vi "解析坐标.vi"(8 "线号":string, 10 "匹配字符":string="J", 11 "解析数组":string[](array[string])) -> (1 "编码数值":i32, 2 "进出线选项":T1, 3 "坐标xy顺序":string[](array[string]))   [LabVIEW 2014]
uses:
  Global.vi
  <vilib>/vision/NI_Vision_Development_Module.lvlib
panel:
  out "数组":string[](array[string])
  out "数组输出 2":string[](array[string])
  out "数组输出":string[](array[string])
  out "x >= 0?":bool
  # "第二象限顺/逆"
  # "第一象限顺/逆"
  # "第三象限顺/逆"
  # "第四象限顺/逆"
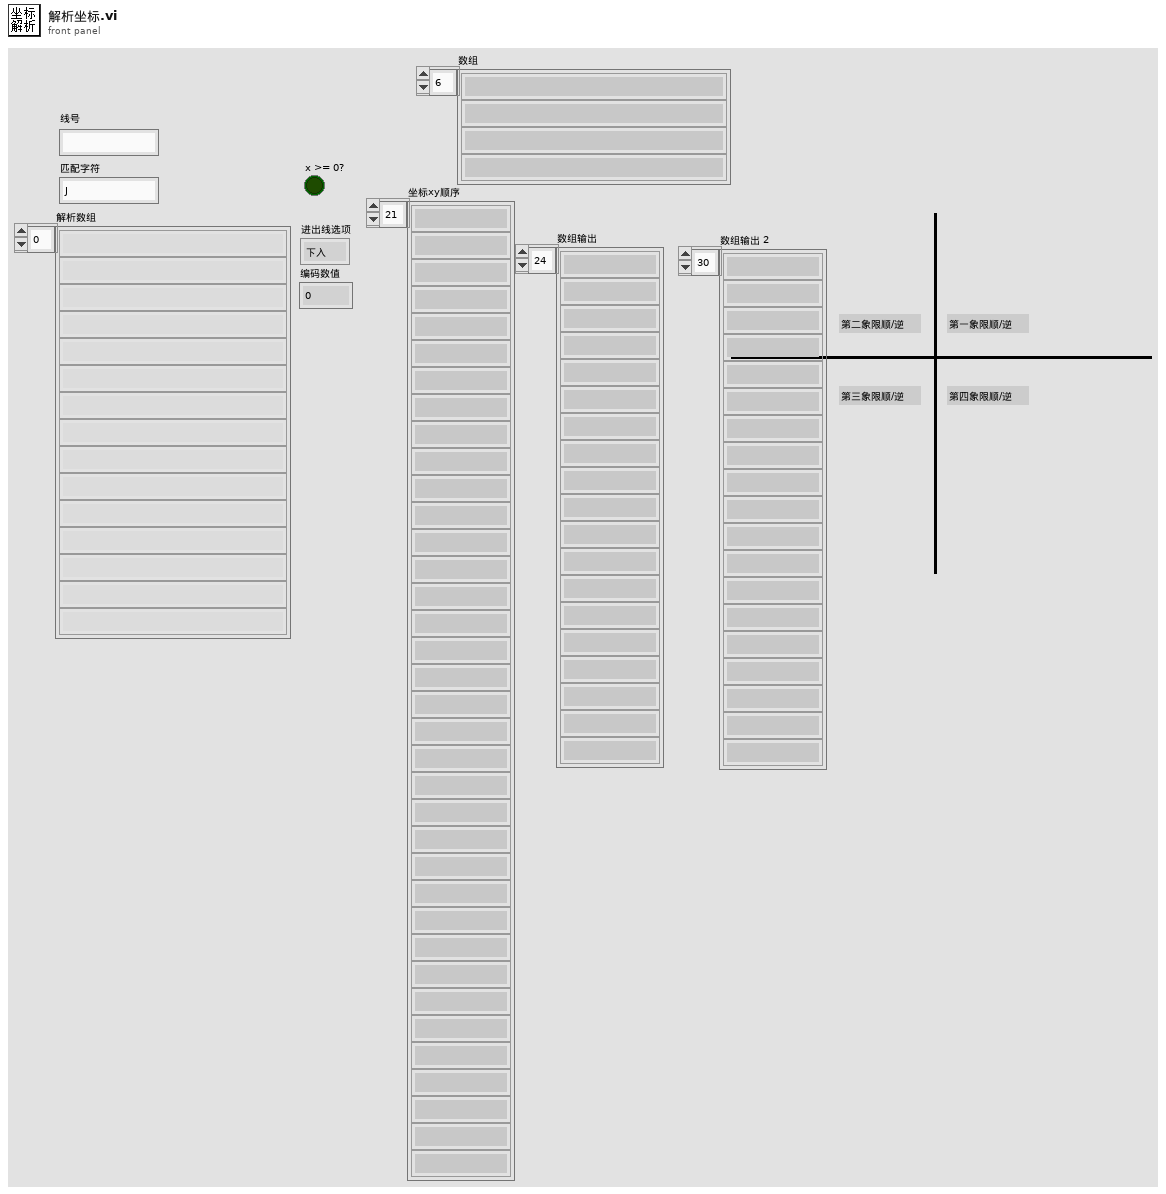
[diagram p1: front panel]
types:
  T1 = typedef "进出线选项.ctl" = enum16{"下入", "上入", "下出", "上出"}
  T2 = cluster{"Center":cluster{"X":sgl, "Y":sgl}, "Radius":dbl}
  T3 = typedef "XYPos.ctl" = cluster{"X":dbl, "Y":dbl}
  T4 = typedef "mark规格.ctl" = cluster{"X下限":dbl, "X上限":dbl, "Y下限":dbl, "Y 上限":dbl, "angle下限":dbl, "angle上限":dbl}
  T5 = cluster{"甩线补偿值":cluster{"下边":dbl, "距离上边":dbl, "左边":dbl, "右边":dbl}, "补偿甩线坐标偏移":T3, "mark点模组补偿":T3, "出线补偿值":dbl, "mark规格":T4}
  T6 = cluster{"下边":dbl, "距离上边":dbl, "左边":dbl, "右边":dbl}
  T7 = cluster{"result string":dbl, "result string":dbl}
  T8 = cluster{"result string":dbl, "result string":dbl}[]
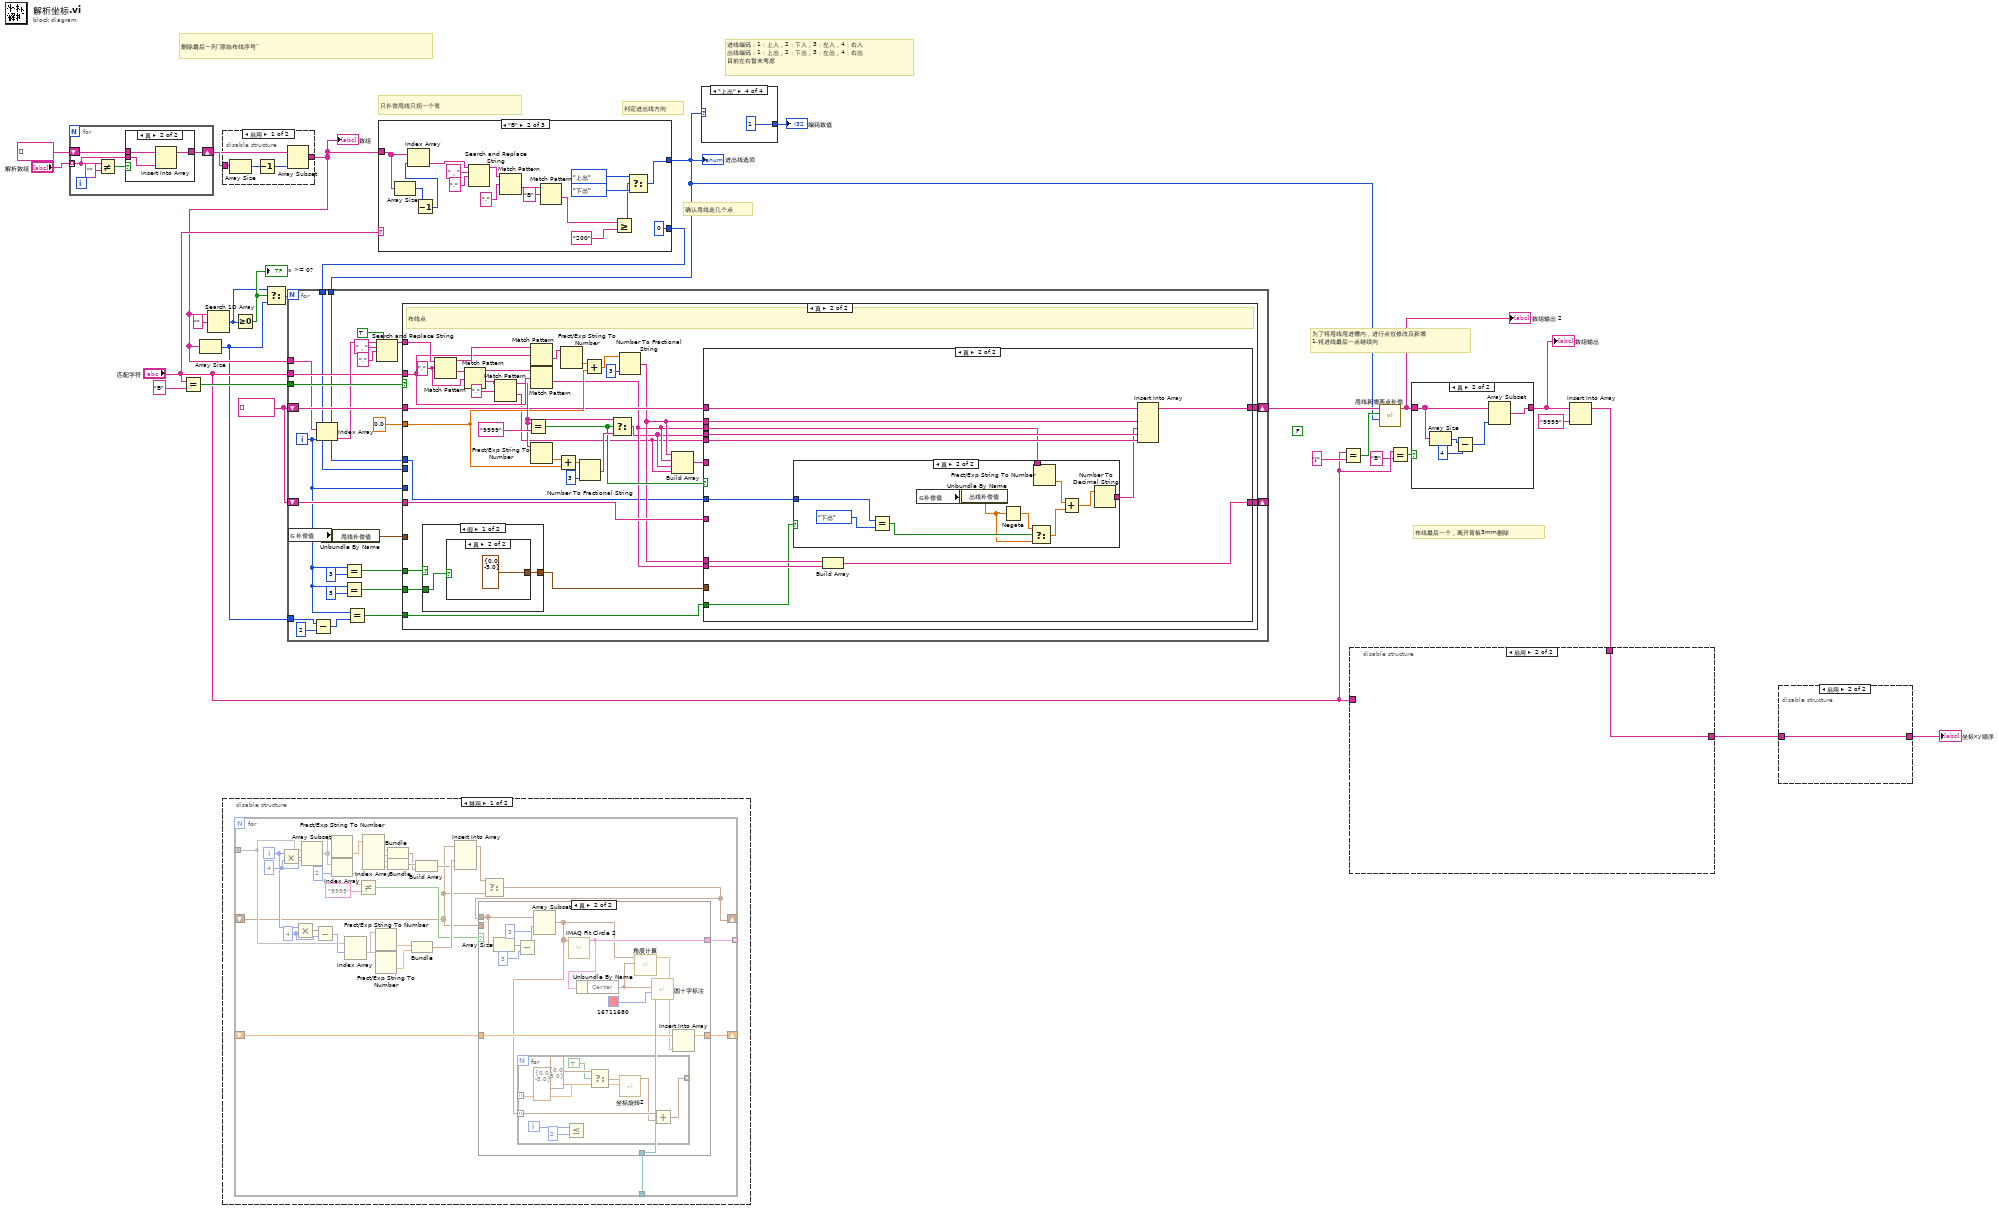
[diagram p0: block diagram]
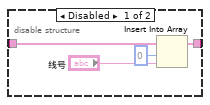
[diagram p3: hidden frame]
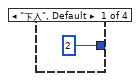
[diagram p5: hidden frame]
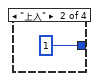
[diagram p6: hidden frame]
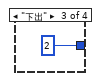
[diagram p7: hidden frame]
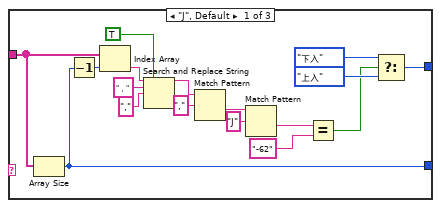
[diagram p8: hidden frame]
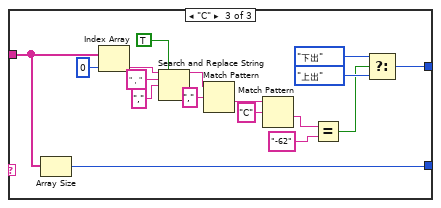
[diagram p9: hidden frame]
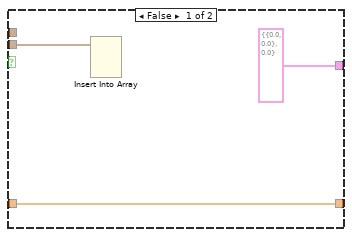
[diagram p11: hidden frame]
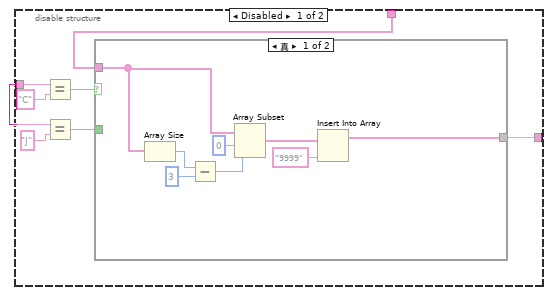
[diagram p13: hidden frame]
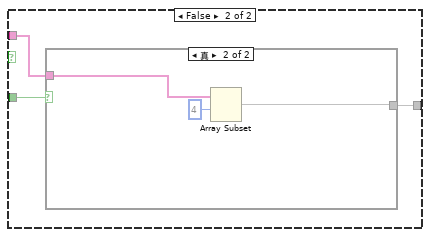
[diagram p14: hidden frame]
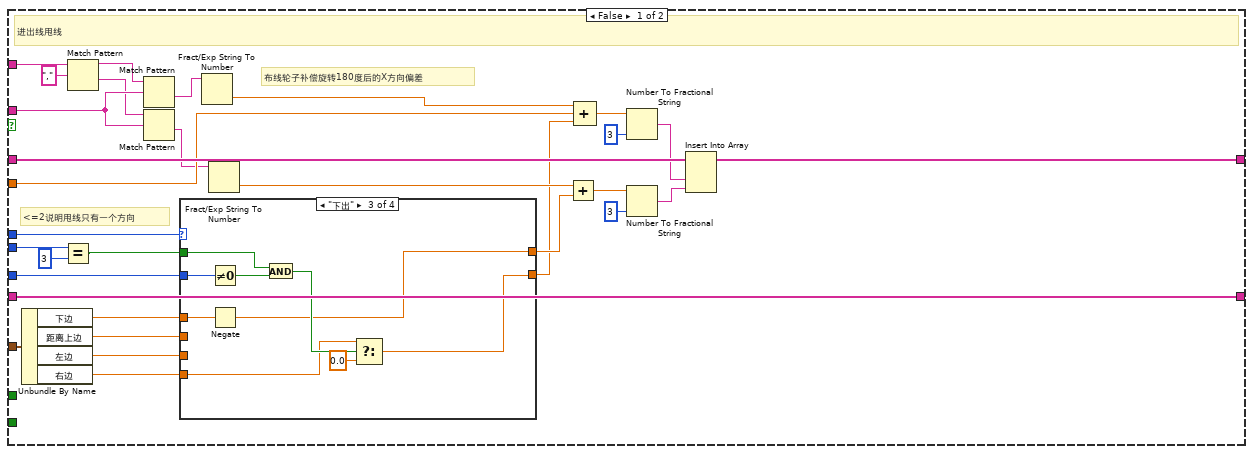
[diagram p16: hidden frame]
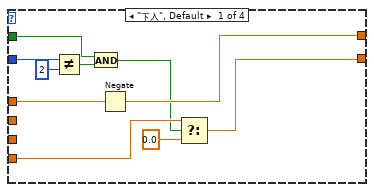
[diagram p17: hidden frame]
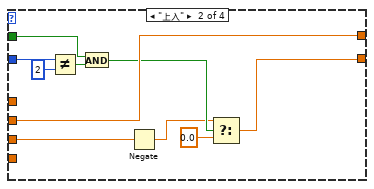
[diagram p18: hidden frame]
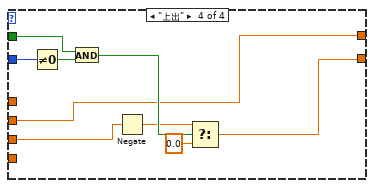
[diagram p19: hidden frame]
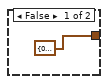
[diagram p20: hidden frame]
diagram:
  (unwired) FALSE
  w19 = string[] []
  # "删除最后一列“原始布线序号”"
  # "布线最后一个，离开背板3mm删除"
  # "为了将甩线甩进槽内，进行点位修改及新增\n1.将进线最后一点继续向"
  # "进线编码：1：上入，2：下入，3：左入，4：右入\n出线编码：1：上出，2：下出，3：左出，4：右出\n目前左右暂未考虑"
  # "确认甩线走几个点"
  # "判定进出线方向"
  # "只补偿甩线只拐一个弯"
  n1 = for {
    tunnel: "解析数组" -> [w28] mode=indexing
    shift-right: [w31] -> w5
    shift-left: string[] [] -> [w32]
    n2 = Not Equal?(x=w28, y="") -> (x != y?=w29:bool)
    n3 = case shown="真" w29 {
      tunnel: w32 -> [w33 w36]
      tunnel: [w33 w35] -> w31
      tunnel: w28 -> [_ w34]
      frame False {
      }
      frame True {
        n4 = Insert Into Array(array=w36, new element=w34) -> (w35:string[])  [unwired: 1 in]
      }
    }
  }
  n5 = Equal?(x="匹配字符", y="B") -> (x = y?=w26:bool)
  n6 = disable-structure shown="启用" {
    disable-tunnel: w5 -> [w40 w41]
    disable-tunnel: [w39 w41] -> w4
    frame Enabled {
      n7 = Array Size(array=w40) -> (size(s)=w38:i32)
      n8 = Decrement(x=w38) -> (x-1=w37:i32)
      n9 = Array Subset(array=w40, length=w37) -> (w39:string[])  [unwired: 1 in]
    }
    frame Disabled {
    }
  }
  "数组" <- w4
  n10 = Array Size(array=w4) -> (size(s)=w1:i32)
  n11 = Search 1D Array(1D array=w4, element="" ("元素")) -> (index of element=w23:i32)  [unwired: 1 in]
  n12 = disable-structure shown="禁用" {
    frame Disabled {
      n13 = for {
        tunnel: _ -> [w51]
        shift-right: [w46] -> _
        shift-left: _ -> [w42]
        tunnel: [w48] -> _ mode=indexing
        tunnel: _ -> [w45]
        shift-right: [w43] -> _
        shift-left: _ -> [w44]
        i -> [w52]
        w55 = 4 ("y")
        w72 = 4 ("y")
        n14 = Multiply(x=w52, y=w72) -> (x*y=w73:i32)
        n15 = Multiply(x=w52, y=w55) -> (x*y=w53:i32)
        n16 = Array Subset(array=w51, index=w73, length=w72) -> (w67:void[])
        n17 = Subtract(x=w53, y=w55) -> (x-y=w54:i32)
        n18 = Fract/Exp String To Number(string=w67) -> (number=w64:dbl[])  [unwired: 3 in, 1 out]
        n19 = Index Array(array=w67, index=2 ("索引")) -> (element=w70)
        n20 = Index Array(array=w51, index #1=w54) -> (element #1=w57, element #2=w58)  [unwired: 1 in]
        n21 = Not Equal?(x=w70, y="9999") -> (x != y?=w47:bool)
        n22 = Index Array(array=w64) -> (element #1=w66:dbl, element #2=w65:dbl, element #3=w63:dbl, element #4=w62:dbl)  [unwired: 4 in]
        n23 = Fract/Exp String To Number(string=w57) -> (number=w56:dbl)  [unwired: 3 in, 1 out]
        n24 = Fract/Exp String To Number(string=w58) -> (number=w59:dbl)  [unwired: 3 in, 1 out]
        n25 = Bundle(w66, w65) -> (w60:cluster{dbl, dbl})  [unwired: 1 in]
        n26 = Bundle(w63, w62) -> (w61:cluster{dbl, dbl})  [unwired: 1 in]
        n27 = Bundle(w56, w59) -> (w50:cluster{dbl, dbl})  [unwired: 1 in]
        n28 = Build Array(w61, w60) -> (w49:cluster{dbl, dbl}[])
        n29 = Insert Into Array(array=w42, new element #1=w50, new element #2=w49) -> (w68:cluster{dbl, dbl}[])  [unwired: 1 in]
        n30 = Select(t=w68, f=w42) -> (s? t:f=w46:cluster{dbl, dbl}[])  [unwired: 1 in]
        n31 = case shown="真" w47 {
          tunnel: [T2 {"Center"={"X"=0.0, "Y"=0.0}, "Radius"=0.0} ("Circle") w83] -> w48
          tunnel: w46 -> [_ w89]
          tunnel: w45 -> [_ w84]
          tunnel: w44 -> [w75 w80]
          tunnel: [w75 w79] -> w43
          tunnel: w42 -> [w74 _]
          frame False {
            n32 = Insert Into Array(array=w74) -> ()  [unwired: 3 in, 1 out]
          }
          frame True {
            n33 = Array Size(array=w89) -> (size(s)=w88:i32)
            n34 = Subtract(x=w88, y=3) -> (x-y=w86:i32)
            n35 = Array Subset(array=w89, index=w86, length=3 ("长度")) -> (w77:cluster{dbl, dbl}[])
            n36 = for {
              tunnel: w77 -> [w98] mode=indexing
              tunnel: _ -> [w99] mode=indexing
              tunnel: [w96] -> _ mode=indexing
              i -> [w95]
              n37 = Less Or Equal?(x=w95, y=2) -> ()  [unwired: 1 out]
              n38 = Select(t=cluster{"X":dbl, "Y":dbl} {"X"=0.0, "Y"=5.0} ("y"), s=TRUE, f=cluster{"X":dbl, "Y":dbl} {"X"=0.0, "Y"=-5.0} ("y")) -> (s? t:f=w92:cluster{"X":dbl, "Y":dbl})
              n39 = call "坐标旋转2.vi"("旋转角度(单位弧度)"=w99, "dtx,dty In"=w92) -> ("dtx,dty Out"=w97:cluster{"X":dbl, "Y":dbl})  [unwired: 9 in]
              n40 = Add(x=w98, y=w97) -> (x+y=w96:cluster{dbl, dbl})
            }
            n41 = call "IMAQ Fit Circle 2"("Radial Points"=w77) -> ("Circle"=w83:T2)  [unwired: 5 in, 5 out]
            n42 = Unbundle By Name(w83) -> ("Center"=w81:cluster{"X":sgl, "Y":sgl})
            n43 = call "角度计算.vi"("远心坐标"=w81, "圆弧上三个点坐标"=w77) -> ("Angle"=w78:dbl[])  [unwired: 9 in]
            n44 = call "圆十字标注.vi"("Color"=u32 16711680, "簇"=w81, "引用句柄输入"=w84) -> ()  [unwired: 8 in, 1 out]
            n45 = Insert Into Array(array=w80, new element=w78) -> (w79:dbl[])  [unwired: 1 in]
          }
        }
      }
    }
    frame Enabled {
    }
  }
  n46 = Greater Or Equal To 0?(x=w23) -> (x >= 0?=w24:bool)
  "x >= 0?" <- w24
  n47 = Select(t=w23, s=w24, f=w1) -> (s? t:f=w22:i32)
  n48 = case shown="\"B\"" "匹配字符" {
    tunnel: w4 -> [w107 w128 w150]
    tunnel: [w103 w120 w139] -> w11
    tunnel: [w100 0 w135] -> w16
    frame "J", Default {
      n49 = Array Size(array=w107) -> (size(s)=w100:i32)
      n50 = Decrement(x=w100) -> (x-1=w116:i32)
      n51 = Index Array(array=w107, index=w116) -> (element=w113:string)
      n52 = Search and Replace String(replace all?=TRUE ("替换全部？(F)"), input string=w113, search string="，" ("搜索字符串"), replace string="," ("替换字符串(\"\")")) -> (result string=w111:string)  [unwired: 4 in, 3 out]
      n53 = Match Pattern(string=w111, regular expression="," ("正则表达式")) -> (after substring=w109:string)  [unwired: 1 in, 3 out]
      n54 = Match Pattern(string=w109, regular expression="J" ("正则表达式")) -> (after substring=w101:string)  [unwired: 1 in, 3 out]
      n55 = Equal?(x=w101, y="-62") -> (x = y?=w102:bool)
      n56 = Select(t=进出线选项."下入", s=w102, f=进出线选项."上入") -> (s? t:f=w103:T1)
    }
    frame "B" {
      n57 = Array Size(array=w128) -> (size(s)=w118:i32)
      n58 = Decrement(x=w118) -> (x-1=w117:i32)
      n59 = Index Array(array=w128, index=w117) -> (element=w127:string)
      n60 = Search and Replace String(input string=w127, search string="，" ("搜索字符串"), replace string="," ("替换字符串(\"\")")) -> (result string=w125:string)  [unwired: 5 in, 3 out]
      n61 = Match Pattern(string=w125, regular expression="," ("正则表达式")) -> (after substring=w130:string)  [unwired: 1 in, 3 out]
      n62 = Match Pattern(string=w130, regular expression="B" ("正则表达式")) -> (after substring=w119:string)  [unwired: 1 in, 3 out]
      n63 = Greater Or Equal?(x=w119, y="200") -> (x >= y?=w121:bool)
      n64 = Select(t=进出线选项."上出", s=w121, f=进出线选项."下出") -> (s? t:f=w120:T1)
    }
    frame "C" {
      n65 = Array Size(array=w150) -> (size(s)=w135:i32)
      n66 = Index Array(array=w150, index=0 ("索引")) -> (element=w147:string)
      n67 = Search and Replace String(replace all?=TRUE ("替换全部？(F)"), input string=w147, search string="，" ("搜索字符串"), replace string="," ("替换字符串(\"\")")) -> (result string=w145:string)  [unwired: 4 in, 3 out]
      n68 = Match Pattern(string=w145, regular expression="," ("正则表达式")) -> (after substring=w143:string)  [unwired: 1 in, 3 out]
      n69 = Match Pattern(string=w143, regular expression="C" ("正则表达式")) -> (after substring=w137:string)  [unwired: 1 in, 3 out]
      n70 = Equal?(x=w137, y="-62") -> (x = y?=w136:bool)
      n71 = Select(t=进出线选项."下出", s=w136, f=进出线选项."上出") -> (s? t:f=w139:T1)
    }
  }
  "进出线选项" <- w11
  n72 = for {
    N: w22 -> [_]
    tunnel: w4 -> [w167]
    tunnel: "匹配字符" -> [w168]
    shift-right: [w175] -> w13
    shift-left: w19 -> [w176]
    tunnel: w26 -> [w174]
    shift-right: [w165] -> _
    shift-left: w19 -> [w166]
    tunnel: w11 -> [w160]
    tunnel: w16 -> [w159]
    tunnel: w1 -> [w155]
    i -> [w157]
    n73 = global read "Global.vi" "补偿值"() -> (w152:T5)
    n74 = Subtract(x=w155, y=2) -> (x-y=w154:i32)
    n75 = Index Array(array=w167, index=w157) -> (element=w169:string)
    n76 = Unbundle By Name(w152) -> ("甩线补偿值"=w151:T6)
    n77 = Equal?(x=w157, y=3) -> (x = y?=w163:bool)
    n78 = Equal?(x=w157, y=5) -> (x = y?=w161:bool)
    n79 = Equal?(x=w157, y=w154) -> (x = y?=w156:bool)
    n80 = Search and Replace String(replace all?=TRUE ("替换全部？(F)"), input string=w169, search string="，" ("搜索字符串"), replace string="," ("替换字符串(\"\")")) -> (result string=w171:string)  [unwired: 4 in, 3 out]
    n81 = case shown="真" w174 {
      tunnel: w168 -> [w207 w272]
      tunnel: w171 -> [w206 w279]
      tunnel: w176 -> [w202 w255]
      tunnel: [w177 w256] -> w175
      tunnel: 0.0 -> [w197 w261]
      tunnel: w166 -> [w195 w258]
      tunnel: [w195 w259] -> w165
      tunnel: w163 -> [_ w250]
      tunnel: w161 -> [_ w249]
      tunnel: w151 -> [w189 _]
      tunnel: w160 -> [w188 w247]
      tunnel: w159 -> [w180 _]
      tunnel: w157 -> [w183 _]
      tunnel: w156 -> [_ w246]
      frame False {
        # "<=2说明甩线只有一个方向"
        # "布线轮子补偿旋转180度后的X方向偏差"
        # "进出线甩线"
        n82 = Unbundle By Name(w189) -> ("下边"=w187:dbl, "距离上边"=w186:dbl, "左边"=w185:dbl, "右边"=w184:dbl)
        n83 = Equal?(x=w180, y=3) -> (x = y?=w178:bool)
        n84 = Match Pattern(string=w206, regular expression="," ("正则表达式")) -> (before substring=w204:string, after substring=w203:string)  [unwired: 1 in, 2 out]
        n85 = Match Pattern(string=w204, regular expression=w207) -> (after substring=w196:string)  [unwired: 1 in, 3 out]
        n86 = Match Pattern(string=w203, regular expression=w207) -> (after substring=w191:string)  [unwired: 1 in, 3 out]
        n87 = case shown="\"下出\"" w188 {
          tunnel: w178 -> [w210 w221 w230 w237]
          tunnel: w187 -> [w217 _ w231 _]
          tunnel: w186 -> [_ w226 _ w240]
          tunnel: w185 -> [_ w224 _ w242]
          tunnel: w184 -> [w213 _ w235 _]
          tunnel: w183 -> [w209 w219 w229 w239]
          tunnel: [w216 w226 w232 w240] -> w182
          tunnel: [w215 w227 w233 w243] -> w181
          frame "下入", Default {
            n88 = Not Equal?(x=w209, y=2 ("x")) -> (x != y?=w214:bool)
            n89 = And(x=w210, y=w214) -> (x .and. y?=w211:bool)
            n90 = Negate(x=w217) -> (-x=w216:dbl)
            n91 = Select(t=w213, s=w211, f=0.0 ("t")) -> (s? t:f=w215:dbl)
          }
          frame "上入" {
            n92 = Not Equal?(x=w219, y=2 ("x")) -> (x != y?=w218:bool)
            n93 = And(x=w221, y=w218) -> (x .and. y?=w225:bool)
            n94 = Negate(x=w224) -> (-x=w222:dbl)
            n95 = Select(t=w222, s=w225, f=0.0 ("t")) -> (s? t:f=w227:dbl)
          }
          frame "下出" {
            n96 = Not Equal To 0?(x=w229) -> (x != 0?=w228:bool)
            n97 = Negate(x=w231) -> (-x=w232:dbl)
            n98 = And(x=w230, y=w228) -> (x .and. y?=w236:bool)
            n99 = Select(t=w235, s=w236, f=0.0) -> (s? t:f=w233:dbl)
          }
          frame "上出" {
            n100 = Not Equal To 0?(x=w239) -> (x != 0?=w238:bool)
            n101 = And(x=w237, y=w238) -> (x .and. y?=w245:bool)
            n102 = Negate(x=w242) -> (-x=w241:dbl)
            n103 = Select(t=w241, s=w245, f=0.0) -> (s? t:f=w243:dbl)
          }
        }
        n104 = Fract/Exp String To Number(string=w196) -> (number=w201:dbl)  [unwired: 3 in, 1 out]
        n105 = Fract/Exp String To Number(string=w191) -> (number=w192:dbl)  [unwired: 3 in, 1 out]
        n106 = Add(x=w192, y=w182) -> (x+y=w193:dbl)
        n107 = Compound Arithmetic op=ADD(w201, w197, w181) -> (w200:dbl)
        n108 = Number To Fractional String(number=w200, precision (6)=i16 3 ("精度(6)")) -> (F-format string=w198:string)  [unwired: 2 in]
        n109 = Number To Fractional String(number=w193, precision (6)=i16 3 ("精度(6)")) -> (F-format string=w190:string)  [unwired: 2 in]
        n110 = Insert Into Array(array=w202, new element #1=w198, new element #2=w190) -> (w177:string[])  [unwired: 1 in]
      }
      frame True {
        w276 = "," ("正则表达式")
        # "布线点"
        n111 = case shown="假" w250 {
          tunnel: w249 -> [w281 _]
          tunnel: [w280 cluster{"X":dbl, "Y":dbl} {"X"=0.0, "Y"=5.0} ("y")] -> w248
          frame False {
            n112 = case shown="真" w281 {
              tunnel: [cluster{"X":dbl, "Y":dbl} {"X"=0.0, "Y"=-5.0} ("y") cluster{"X":dbl, "Y":dbl} {"X"=0.0, "Y"=-5.0} ("y")] -> w280
              frame False {
              }
              frame True {
              }
            }
          }
          frame True {
          }
        }
        n113 = Match Pattern(string=w279, regular expression=w276) -> (before substring=w274:string, after substring=w278:string)  [unwired: 1 in, 2 out]
        n114 = Match Pattern(string=w278, regular expression=w276) -> (before substring=w273:string, after substring=w277:string)  [unwired: 1 in, 2 out]
        n115 = Match Pattern(string=w277, regular expression="," ("正则表达式")) -> (before substring=w263:string, after substring=w251:string)  [unwired: 1 in, 2 out]
        n116 = Equal?(x=w263, y="9999") -> (x = y?=w260:bool)
        n117 = Match Pattern(string=w274, regular expression=w272) -> (after substring=w271:string)  [unwired: 1 in, 3 out]
        n118 = Match Pattern(string=w273, regular expression=w272) -> (after substring=w253:string)  [unwired: 1 in, 3 out]
        n119 = Fract/Exp String To Number(string=w263) -> (number=w264:dbl)  [unwired: 3 in, 1 out]
        n120 = Add(x=w264, y=w261) -> (x+y=w265:dbl)
        n121 = Fract/Exp String To Number(string=w271) -> (number=w270:dbl)  [unwired: 3 in, 1 out]
        n122 = Number To Fractional String(number=w265, precision (6)=i16 3 ("精度(6)")) -> (F-format string=w262:string)  [unwired: 2 in]
        n123 = Add(x=w270, y=w261) -> (x+y=w269:dbl)
        n124 = Select(t=w263, s=w260, f=w262) -> (s? t:f=w252:string)
        n125 = Number To Fractional String(number=w269, precision (6)=i16 3 ("精度(6)")) -> (F-format string=w254:string)  [unwired: 2 in]
        n126 = Build Array(w254, w253, w252, w251) -> (w257:string[])
        n127 = case shown="真" w260 {
          tunnel: w254 -> [_ w362]
          tunnel: w253 -> [_ w361]
          tunnel: [w292 w360] -> w259
          tunnel: w258 -> [w292 _]
          tunnel: w257 -> [w293 _]
          tunnel: [w291 w358] -> w256
          tunnel: w255 -> [w290 w359]
          tunnel: w254 -> [w288 w357]
          tunnel: w253 -> [w287 w354]
          tunnel: w252 -> [w286 w356]
          tunnel: w251 -> [w285 w355]
          tunnel: w248 -> [w289 _]
          tunnel: w247 -> [_ w353]
          tunnel: w246 -> [_ w351]
          frame False {
            n128 = disable-structure shown="启用" {
              disable-tunnel: w293 -> [w317 _]
              disable-tunnel: w292 -> [w308 _]
              disable-tunnel: [w307 w349] -> w291
              disable-tunnel: w290 -> [w297 w350]
              disable-tunnel: w289 -> [w294 _]
              disable-tunnel: w288 -> [_ w348]
              disable-tunnel: w287 -> [_ w345]
              disable-tunnel: w286 -> [_ w347]
              disable-tunnel: w285 -> [_ w346]
              frame Disabled {
                n129 = Fract/Exp String To Number(string=w317) -> (number=w320:dbl[])  [unwired: 3 in, 1 out]
                n130 = Fract/Exp String To Number(string=w308) -> (number=w315:dbl[])  [unwired: 3 in, 1 out]
                n131 = Index Array(array=w320) -> (element #1=w318:dbl, element #2=w319:dbl, element #3=w321:dbl, element #4=w316:dbl)  [unwired: 4 in]
                n132 = Index Array(array=w315) -> (element #1=w314:dbl, element #2=w313:dbl)  [unwired: 2 in]
                n133 = Bundle("result string"=w318, "result string"=w319) -> (w305:T7)  [unwired: 1 in]
                n134 = Bundle("result string"=w321, "result string"=w316) -> (w304:T7)  [unwired: 1 in]
                n135 = Bundle(w314, w313) -> (w306:cluster{dbl, dbl})  [unwired: 1 in]
                n136 = Build Array(w304, w305, w306) -> (w309:T8)
                n137 = Build Array(w306, w305, w304) -> (w303:T8)
                n138 = call "IMAQ Fit Circle 2"("Radial Points"=w309) -> ("Circle"=w312:T2)  [unwired: 5 in, 5 out]
                n139 = Unbundle By Name(w312) -> ("Center"=w311:cluster{"X":sgl, "Y":sgl})
                n140 = call "角度计算.vi"("远心坐标"=w311, "圆弧上三个点坐标"=w303) -> ("Angle"=w310:dbl[])  [unwired: 9 in]
                n141 = for {
                  tunnel: w310 -> [w335] mode=indexing
                  tunnel: [w330] -> _ mode=indexing
                  tunnel: w303 -> [w333] mode=indexing
                  shift-right: [w325] -> w299
                  shift-left: string[] [] -> [w331]
                  tunnel: w294 -> [w322]
                  i -> [w326]
                  n142 = call "坐标旋转2.vi"("旋转角度(单位弧度)"=w335, "dtx,dty In"=w322) -> ("dtx,dty Out"=w334:cluster{"X":dbl, "Y":dbl})  [unwired: 9 in]
                  n143 = Add(x=w333, y=w334) -> (x+y=w330:cluster{dbl, dbl})
                  n144 = Number To Fractional String(number=w330, precision (6)=i16 3 ("精度(6)")) -> (F-format string=w329:cluster{string, string})  [unwired: 2 in]
                  n145 = Equal To 0?(x=w326) -> (x = 0?=w324:bool)
                  n146 = Unbundle(w329) -> (w328:string, w327:string)
                  n147 = case shown="真" w324 {
                    tunnel: w331 -> [w339 w344]
                    tunnel: w328 -> [w337 w343]
                    tunnel: w327 -> [w336 w342]
                    tunnel: [w338 w341] -> w325
                    tunnel: "9999" -> [_ w340]
                    frame False {
                      n148 = Insert Into Array(array=w339, new element #1=w337, new element #2=w336) -> (w338:string[])  [unwired: 1 in]
                    }
                    frame True {
                      n149 = Insert Into Array(array=w344, new element #1=w343, new element #2=w342, new element #3=w340, new element #4=w340) -> (w341:string[])  [unwired: 1 in]
                    }
                  }
                }
                n150 = Array Size(array=w297) -> (size(s)=w302:i32)
                n151 = Subtract(x=w302, y=4) -> (x-y=w296:i32)
                n152 = Delete From Array(array=w297, length=4 ("长度"), index=w296) -> (array with subset deleted=w298:string[])  [unwired: 1 out]
                n153 = Insert Into Array(array=w298, new element=w299) -> (w307:string[])  [unwired: 1 in]
              }
              frame Enabled {
                n154 = Insert Into Array(array=w350, new element #1=w348, new element #2=w345, new element #3=w347, new element #4=w346) -> (w349:string[])  [unwired: 1 in]
              }
            }
          }
          frame True {
            n155 = case shown="真" w351 {
              tunnel: w354 -> [w363 w374]
              tunnel: w353 -> [_ w373]
              tunnel: [w363 w366] -> w352
              frame False {
              }
              frame True {
                n156 = Equal?(x=w373, y=进出线选项."下出") -> (x = y?=w368:bool)
                n157 = global read "Global.vi" "补偿值"() -> (w365:T5)
                n158 = Unbundle By Name(w365) -> ("出线补偿值"=w364:dbl)
                n159 = Negate(x=w364) -> (-x=w369:dbl)
                n160 = Select(t=w369, s=w368, f=w364) -> (s? t:f=w370:dbl)
                n161 = Fract/Exp String To Number(string=w374) -> (number=w371:dbl)  [unwired: 3 in, 1 out]
                n162 = Add(x=w371, y=w370) -> (x+y=w367:dbl)
                n163 = Number To Decimal String(number=w367) -> (decimal integer string=w366:string)  [unwired: 1 in]
              }
            }
            n164 = Build Array(w362, w361) -> (w360:string[])
            n165 = Insert Into Array(array=w359, new element #1=w357, new element #2=w352, new element #3=w356, new element #4=w355) -> (w358:string[])  [unwired: 1 in]
          }
        }
      }
    }
  }
  n166 = case shown="\"上出\"" w11 {
    tunnel: [2 1 2 1] -> w15
    frame "下入", Default {
    }
    frame "上入" {
    }
    frame "下出" {
    }
    frame "上出" {
    }
  }
  "编码数值" <- w15
  n167 = Equal?(x="匹配字符", y="J") -> (x = y?=w12:bool)
  n168 = call "甩线新增两点补偿.vi"("进出线选项"=w11, "布尔"=w12, "数组输入"=w13) -> ("数组输出"=w7:string[])  [unwired: 8 in]
  "数组输出 2" <- w7
  n169 = Equal?(x="匹配字符", y="B") -> (x = y?=w8:bool)
  n170 = case shown="真" w8 {
    tunnel: w7 -> [w379 w384]
    tunnel: [w379 w383] -> w6
    frame False {
    }
    frame True {
      n171 = Array Size(array=w384) -> (size(s)=w382:i32)
      n172 = Subtract(x=w382, y=4) -> (x-y=w380:i32)
      n173 = Array Subset(array=w384, length=w380) -> (w383:string[])  [unwired: 1 in]
    }
  }
  "数组输出" <- w6
  n174 = Insert Into Array(array=w6, new element="9999" ("新元素/子数组")) -> (w20:string[])  [unwired: 1 in]
  n175 = disable-structure shown="启用" {
    disable-tunnel: "匹配字符" -> [w386 _]
    disable-tunnel: w20 -> [w389 w407]
    disable-tunnel: [w388 w407] -> w3
    frame Disabled {
      n176 = Equal?(x=w386, y="C") -> (x = y?=w390:bool)
      n177 = Equal?(x=w386, y="J") -> (x = y?=w385:bool)
      n178 = case shown="真" w390 {
        tunnel: w389 -> [w396 w401]
        tunnel: [w397 w400] -> w388
        tunnel: w385 -> [_ w402]
        frame True {
          n179 = Array Size(array=w396) -> (size(s)=w395:i32)
          n180 = Subtract(x=w395, y=3) -> (x-y=w393:i32)
          n181 = Array Subset(array=w396, index=0 ("索引"), length=w393) -> (w398:string[])
          n182 = Insert Into Array(array=w398, new element="9999" ("新元素/子数组")) -> (w397:string[])  [unwired: 1 in]
        }
        frame False {
          n183 = case shown="真" w402 {
            tunnel: w401 -> [w403 w406]
            tunnel: [w403 w404] -> w400
            frame False {
            }
            frame True {
              n184 = Array Subset(array=w406, index=4 ("索引")) -> (w404:string[])  [unwired: 1 in]
            }
          }
        }
      }
    }
    frame Enabled {
    }
  }
  n185 = disable-structure shown="启用" {
    disable-tunnel: w3 -> [w411 w412]
    disable-tunnel: [w410 w412] -> w2
    frame Disabled {
      n186 = Insert Into Array(array=w411, index=0 ("索引"), new element="线号") -> (w410:string[])
    }
    frame Enabled {
    }
  }
  "坐标xy顺序" <- w2
